vi "CmsInitializeDFScript.vi"(8 "error in (no error)":errorcluster) -> (0 "error out":errorcluster, 2 "data event creator":string="CmsDataEventCreator")   [LabVIEW 2017]
uses:
  <vilib>/addons/InsightCM/Devices/Shared/Common/DataFlow/controls/Type.ctl
  <vilib>/addons/InsightCM/Devices/Shared/Cms/CmsAnalysis/CmsAnalysis.lvlib
  <vilib>/addons/InsightCM/Devices/Shared/Common/Trigger/Trigger.lvlib
  <vilib>/addons/InsightCM/Devices/Shared/Common/DataAccumulator/DataAccumulator.lvlib
  <vilib>/addons/InsightCM/Devices/Shared/Cms/CmsVirtualChannel/CmsVirtualChannel.lvlib
  <vilib>/addons/InsightCM/Devices/Shared/Cms/CmsTestPanel/CmsTestPanel.lvlib
  <vilib>/addons/InsightCM/Devices/Shared/Common/DataFlow/DataFlow.lvlib
  <vilib>/addons/InsightCM/Devices/Shared/Common/FileFlow/FileFlow.lvlib
  <vilib>/addons/InsightCM/Devices/Shared/Cms/CmsDataEventCreator/CmsDataEventCreator.lvlib
  <vilib>/addons/InsightCM/Devices/Shared/Common/OpState/OpState.lvlib
  <vilib>/addons/InsightCM/Devices/Shared/Common/TrendAlarm/TrendAlarm.lvlib
  <vilib>/addons/InsightCM/Devices/Shared/Cms/CmsAnalysisHighRate/CmsAnalysisHighRate.lvlib
  <vilib>/addons/InsightCM/Devices/Shared/Cms/CmsBurstMode/BurstMode.lvlib
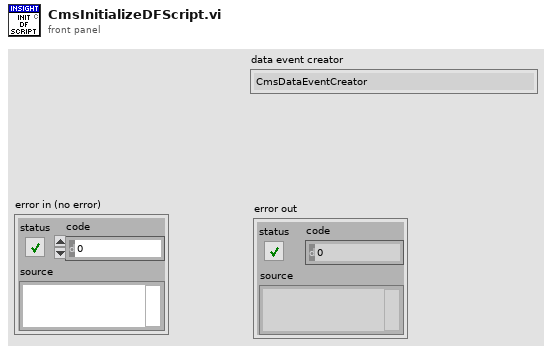
[diagram p1: front panel]
types:
  T1 = typedef "DataFlow.lvlib/Type.ctl" = enum16{"High Rate", "Low Rate", "Burst Mode"}
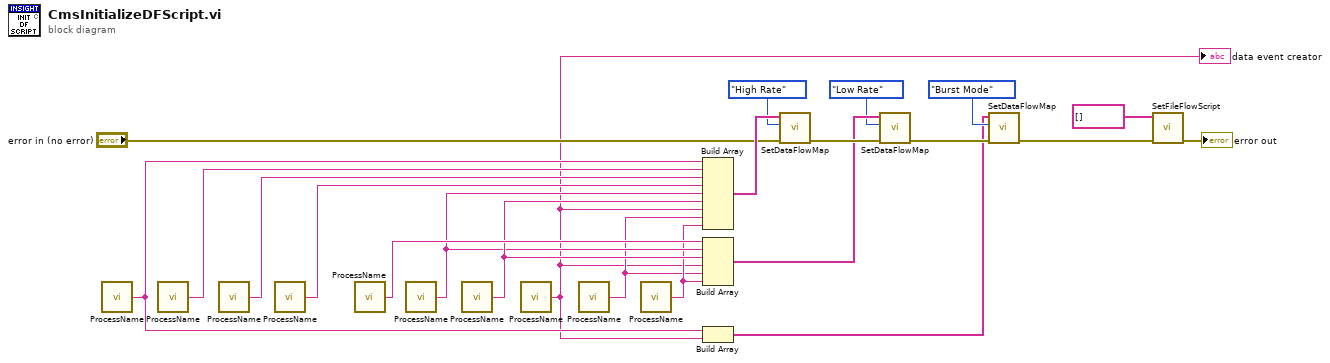
[diagram p0: block diagram]
diagram:
  n1 = call <vilib>:"ProcessName.vi"() -> ("ProcessName"=w3:string)  [unwired: 5 in]
  n2 = call <vilib>:"ProcessName.vi"() -> ("ProcessName"=w12:string)  [unwired: 5 in]
  n3 = call <vilib>:"ProcessName.vi"() -> ("process name"=w13:string)  [unwired: 5 in]
  n4 = call <vilib>:"ProcessName.vi"() -> ("process name"=w11:string)  [unwired: 5 in]
  n5 = call <vilib>:"ProcessName.vi"() -> ("ProcessName"=w17:string)  [unwired: 5 in]
  n6 = call <vilib>:"ProcessName.vi"() -> ("process name"=w14:string)  [unwired: 5 in]
  n7 = call <vilib>:"ProcessName.vi"() -> ("process name"=w15:string)  [unwired: 5 in]
  n8 = call <vilib>:"ProcessName.vi"() -> ("process name"=w2:string)  [unwired: 5 in]
  "data event creator" <- w2
  n9 = call <vilib>:"ProcessName.vi"() -> ("process name"=w7:string)  [unwired: 5 in]
  n10 = call <vilib>:"ProcessName.vi"() -> ("process name"=w8:string)  [unwired: 5 in]
  n11 = Build Array(w3, w12, w13, w11, w14, w15, w2, w7, w8) -> (w22:string[])
  n12 = Build Array(w17, w14, w15, w2, w7, w8) -> (w16:string[])
  n13 = Build Array(w3, w2) -> (w1:string[])
  n14 = call <vilib>:"SetDataFlowMap.vi"("error in (no error)"="error in (no error)", "type"=Type."High Rate", "Dataflow script"=w22) -> ("error out"=w18:errorcluster)  [unwired: 8 in]
  n15 = call <vilib>:"SetDataFlowMap.vi"("error in (no error)"=w18, "type"=Type."Low Rate", "Dataflow script"=w16) -> ("error out"=w5:errorcluster)  [unwired: 8 in]
  n16 = call <vilib>:"SetDataFlowMap.vi"("error in (no error)"=w5, "type"=Type."Burst Mode", "Dataflow script"=w1) -> ("error out"=w4:errorcluster)  [unwired: 8 in]
  n17 = call <vilib>:"SetFileFlowScript.vi"("error in (no error)"=w4, "Fileflow script"=string[] []) -> ("error out"=→"error out":errorcluster)  [unwired: 9 in]
